vi "Read ASIA Global.vi"(8 "error in (no error)":errorcluster, 11 "Pump Number":i32) -> (0 "error out":errorcluster, 3 "Busy":bool)   [LabVIEW 2018, in "ASIA Pump.lvlib"]
uses:
  ASIA Pump.lvlib
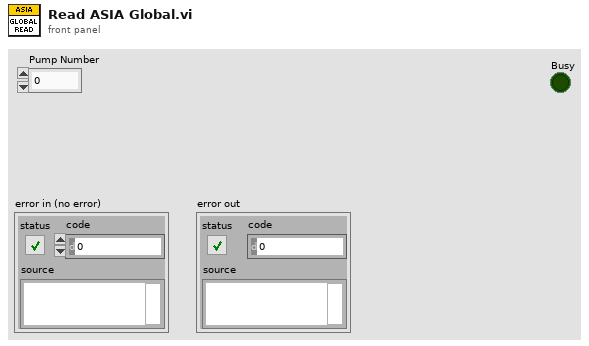
[diagram p1: front panel]
types:
  T1 = cluster{"Busy":bool, "PumpCnt":dbl, "RemoteEntered":bool, "OverpressureSet":bool}[]
  T2 = cluster{"Busy":bool, "PumpCnt":dbl, "RemoteEntered":bool, "OverpressureSet":bool}
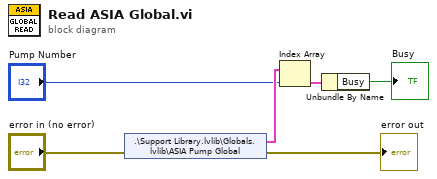
[diagram p0: block diagram]
diagram:
  n1 = shared-variable ".\\Support Library.lvlib\\Globals.lvlib\\ASIA Pump Global"(error in="error in (no error)") -> (w4:T1, error out=→"error out":errorcluster)
  n2 = Index Array(array=w4, index="Pump Number") -> (element=w2:T2)
  n3 = Unbundle By Name(w2) -> ("Busy"=→"Busy":bool)
